vi "Temp.vi"() -> ()   [LabVIEW 2024]
uses:
  <instrlib>/Lake Shore 336/Public/Data/Sensor Data (Single Reading).vi
  <instrlib>/Lake Shore 336/Lake Shore 336.lvlib
panel:
  in  "Stop Button":bool
  out "Sensor D":dbl format="%.3f"
  out "Sensor C":dbl format="%.3f"
  out "Sensor B":dbl format="%.3f"
  out "Sensor A":dbl format="%.3f"
  in  "Lakeshore Temp Controller":refnum<visa-resource-name>
  out "error out":errorcluster
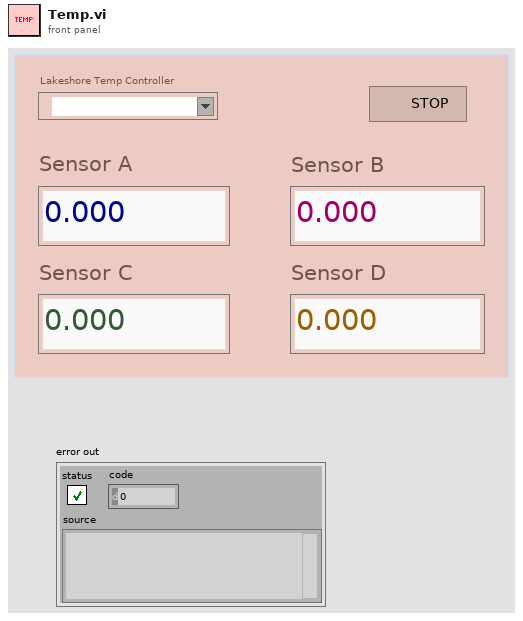
[diagram p1: front panel]
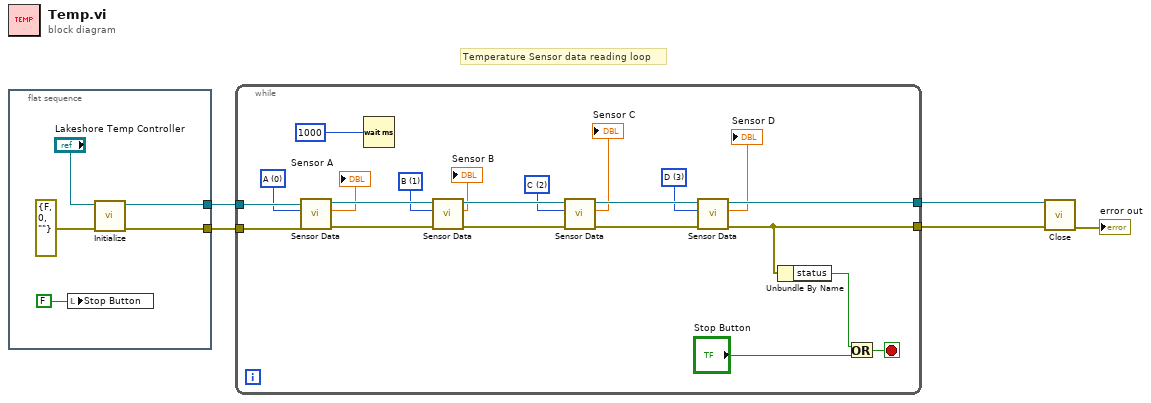
[diagram p0: block diagram]
diagram:
  # "Temperature Sensor data reading loop"
  n1 = flat-sequence {
    tunnel: [w10] -> w5
    tunnel: [w9] -> w4
    frame #0 {
      n2 = local write "Stop Button"(FALSE ("Stop Button")) -> ()
      n3 = call <instrlib>:"Initialize.vi"("error in (no error)"=errorcluster {"status"=FALSE, "code"=0, "source"=""}, "VISA resource name"="Lakeshore Temp Controller") -> ("error out"=w9:errorcluster, "VISA resource name out"=w10:refnum<visa-resource-name>)  [unwired: 8 in]
    }
  }
  n4 = while {
    tunnel: w5 -> [w32]
    tunnel: w4 -> [w31]
    tunnel: [w24] -> w3
    tunnel: [w22] -> w2
    stop <- w21 stop-if-true
    w12 = u16 3 items=["A", "B", "C", "D"] ("Input (0:A)")
    w13 = u16 2 items=["A", "B", "C", "D"] ("Input (0:A)")
    w14 = u16 1 items=["A", "B", "C", "D"] ("Input (0:A)")
    w15 = u16 0 items=["A", "B", "C", "D"] ("Input (0:A)")
    n5 = call-poly <instrlib>:"Sensor Data.vi"("error in (no error)"=w31, "Input (0:A)"=w15, "VISA resource name"=w32) -> ("error out"=w29:errorcluster, "Sensor Data"=→"Sensor A":dbl, "VISA resource name out"=w30:refnum<visa-resource-name>)  [unwired: 6 in]
    n6 = Wait (ms)(milliseconds to wait=u32 1000) -> ()  [unwired: 1 out]
    n7 = call-poly <instrlib>:"Sensor Data.vi"("error in (no error)"=w29, "Input (0:A)"=w14, "VISA resource name"=w30) -> ("error out"=w27:errorcluster, "Sensor Data"=→"Sensor B":dbl, "VISA resource name out"=w28:refnum<visa-resource-name>)  [unwired: 6 in]
    n8 = call-poly <instrlib>:"Sensor Data.vi"("error in (no error)"=w27, "Input (0:A)"=w13, "VISA resource name"=w28) -> ("error out"=w25:errorcluster, "Sensor Data"=→"Sensor C":dbl, "VISA resource name out"=w26:refnum<visa-resource-name>)  [unwired: 6 in]
    n9 = call-poly <instrlib>:"Sensor Data.vi"("error in (no error)"=w25, "Input (0:A)"=w12, "VISA resource name"=w26) -> ("error out"=w22:errorcluster, "Sensor Data"=→"Sensor D":dbl, "VISA resource name out"=w24:refnum<visa-resource-name>)  [unwired: 6 in]
    n10 = Unbundle By Name(w22) -> ("status"=w20:bool)
    n11 = Or(x=w20, y="Stop Button") -> (x .or. y?=w21:bool)
  }
  n12 = call <instrlib>:"Close.vi"("error in (no error)"=w2, "VISA resource name"=w3) -> ("error out"=→"error out":errorcluster)  [unwired: 9 in]
